vi "test.vi"() -> ()   [LabVIEW 2011]
uses:
  functions/Global 2.vi
panel:
  out "Test output":T1
  out "error out":errorcluster
  out "Lines":string[](array[string])
  out "File Status":string
  in  "File Name With Extension":string="test1.cat"
  in  "Path":path=path "C:/Documents and Settings/f100user/My Documents/LabVIEW Data/Script autm"
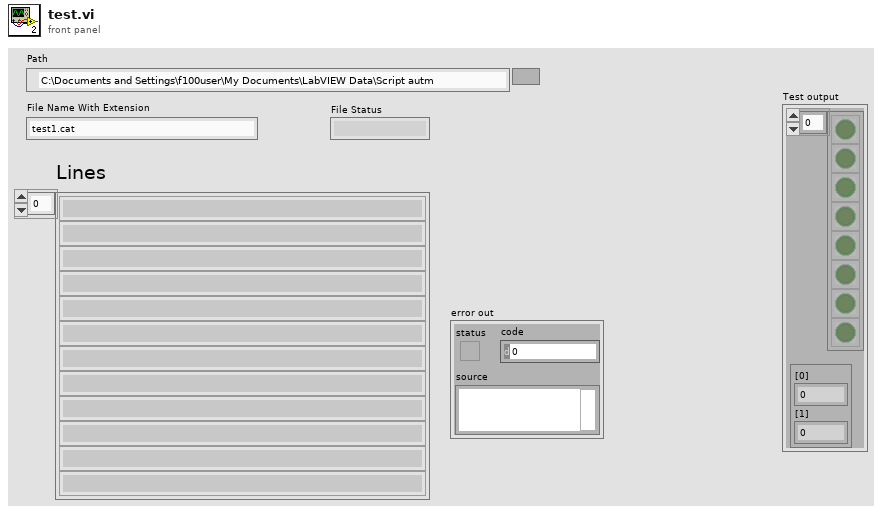
[diagram p1: front panel]
types:
  T1 = cluster{cluster{bool}[], cluster{"[0]":dbl, "[1]":dbl}}
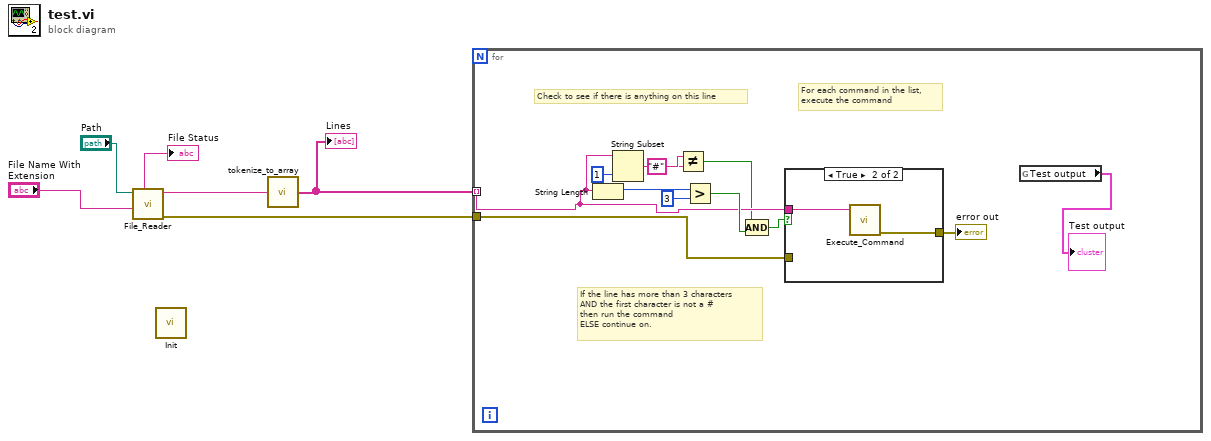
[diagram p0: block diagram]
diagram:
  n1 = call "File_Reader.vi"("File Name With Extension"="File Name With Extension", "Path"="Path") -> ("error out"=w1:errorcluster, "File Contents"=w6:string, "s? t:f"=→"File Status":string)  [unwired: 2 in, 3 out]
  n2 = call "Init.vi"() -> ()  [unwired: 12 in]
  n3 = call "tokenize_to_array.vi"("File Contents"=w6) -> ("Lines"=w2:string[])
  "Lines" <- w2
  n4 = for {
    tunnel: w2 -> [w14] mode=indexing
    tunnel: w1 -> [w8]
    # "If the line has more than 3 characters\nAND the first character is not a #\nthen run the command\nELSE continue on."
    # "Check to see if there is anything on this line"
    # "For each command in the list,\nexecute the command"
    n5 = String Length(string=w14) -> (length=w18:i32)
    n6 = String Subset(string=w14, length (rest)=1 ("length (rest)")) -> (substring=w12:string)  [unwired: 1 out]
    n7 = Not Equal?(x=w12, y="#") -> (x != y?=w10:bool)
    n8 = Greater?(x=w18, y=3) -> (0:w15:bool)
    n9 = Compound Arithmetic op=AND(w10, w15) -> (w16:bool)
    n10 = case shown="True" w16 {
      tunnel: w14 -> [_ w21]
      tunnel: [w19 w20] -> w9
      tunnel: w8 -> [w19 _]
      frame False {
      }
      frame True {
        n11 = call "Execute_Command.vi"("Command"=w21) -> ("error out"=w20:errorcluster)  [unwired: 8 in, 2 out]
      }
    }
    "error out" <- w9
    n12 = global read "Global 2.vi" "Test output"() -> (→"Test output":T1)
  }
